vi "Replace Template Items.vi"(6 "Worker Folder":path, 8 "error in (no error)":errorcluster, 11 "Refs in":T1) -> (0 "error out":errorcluster, 3 "Refs":T1)   [LabVIEW 2020, in "FlexBlocks.lvlib"]
uses:
  FlexBlocks.lvlib
  Scripting Refs.ctl
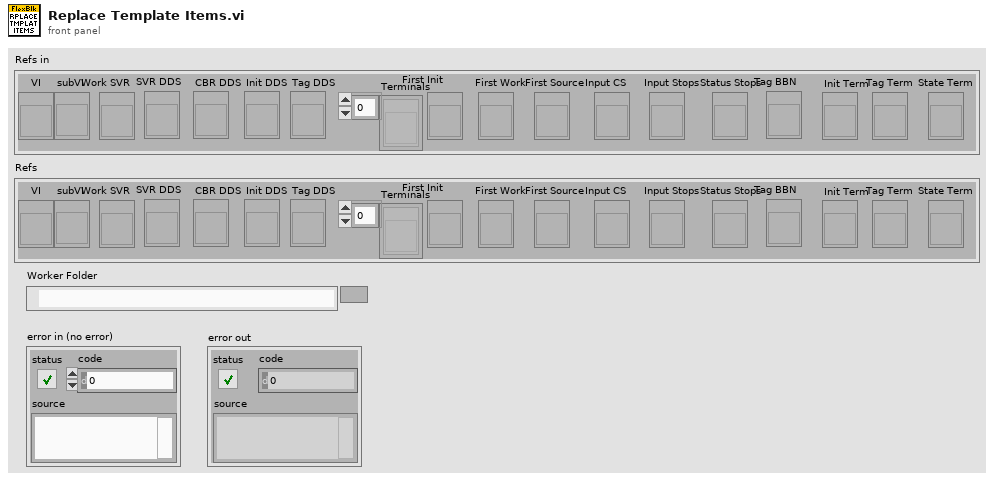
[diagram p1: front panel]
types:
  T1 = typedef "FlexBlocks.lvlib/Scripting Refs.ctl" = cluster{"VI":refnum<vi>, "subVI":refnum<vi>, "Work SVR":refnum<vi>, "SVR DDS":refnum<vi>, "CBR DDS":refnum<vi>, "Init DDS":refnum<vi>, "Tag DDS":refnum<vi>, "Terminals":refnum<vi>[], "First Init":refnum<vi>, "First Work":refnum<vi>, "First Source":refnum<vi>, "Input CS":refnum<vi>, "Input Stops":refnum<vi>, "Status Stops":refnum<vi>, "Tag BBN":refnum<vi>, "Init Term":refnum<vi>, "Tag Term":refnum<vi>, "State Term":refnum<vi>}
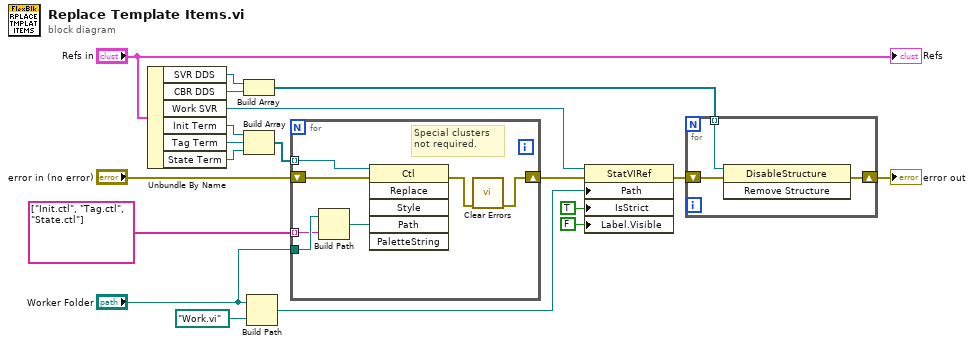
[diagram p0: block diagram]
diagram:
  n1 = Unbundle By Name("Refs in") -> ("SVR DDS"=w3:refnum<vi>, "CBR DDS"=w4:refnum<vi>, "Work SVR"=w6:refnum<vi>, "Init Term"=w8:refnum<vi>, "Tag Term"=w10:refnum<vi>, "State Term"=w9:refnum<vi>)
  n2 = Build Array(w3, w4) -> (w2:refnum<vi>[])
  n3 = Build Array(w8, w10, w9) -> (w7:refnum<vi>[])
  n4 = Build Path(base path="Worker Folder", name or relative path=path "Work.vi") -> (appended path=w15:path)
  n5 = for {
    tunnel: string[] ["Init.ctl", "Tag.ctl", "State.ctl"] -> [w20] mode=indexing
    tunnel: "Worker Folder" -> [w26]
    shift-right: [w23] -> w5
    shift-left: "error in (no error)" -> [w21]
    tunnel: w7 -> [w22] mode=indexing
    # "Special clusters not required."
    n6 = Build Path(base path=w26, name or relative path=w20) -> (appended path=w25:path)
    n7 = invoke class="Ctl" method="Replace"(reference=w22, error in=w21, "Path"=w25) -> (error out=w24:errorcluster)  [unwired: 3 in, 5 out]
    n8 = call <vilib>:"Clear Errors.vi"("error in (no error)"=w24) -> ("error out"=w23:errorcluster)  [unwired: 5 in, 1 out]
  }
  n9 = property class="StatVIRef"(reference=w6, error in=w5, "Path"=w15, "IsStrict"=TRUE ("Is Strict"), "Label.Visible"=FALSE) -> (error out=w13:errorcluster)  [unwired: 1 out]
  n10 = for {
    shift-right: [w29] -> w12
    shift-left: w13 -> [w27]
    tunnel: w2 -> [w28] mode=indexing
    n11 = invoke class="DisableStructure" method="Remove Structure"(reference=w28, error in=w27) -> (error out=w29:errorcluster)  [unwired: 1 in, 2 out]
  }
  "error out" <- w12
  "Refs" <- "Refs in"
